vi "程序选择.vi"() -> ()   [LabVIEW 2018]
panel:
  in  "枚举":enum16{"LABVIEW仿真", "禁用FPGA输入", "使能FPGA输入"}(ring)
  in  "VISA resource name":refnum<visa-resource-name> caption="串口选择"
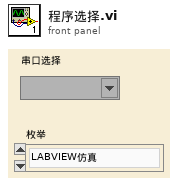
[diagram p1: front panel]
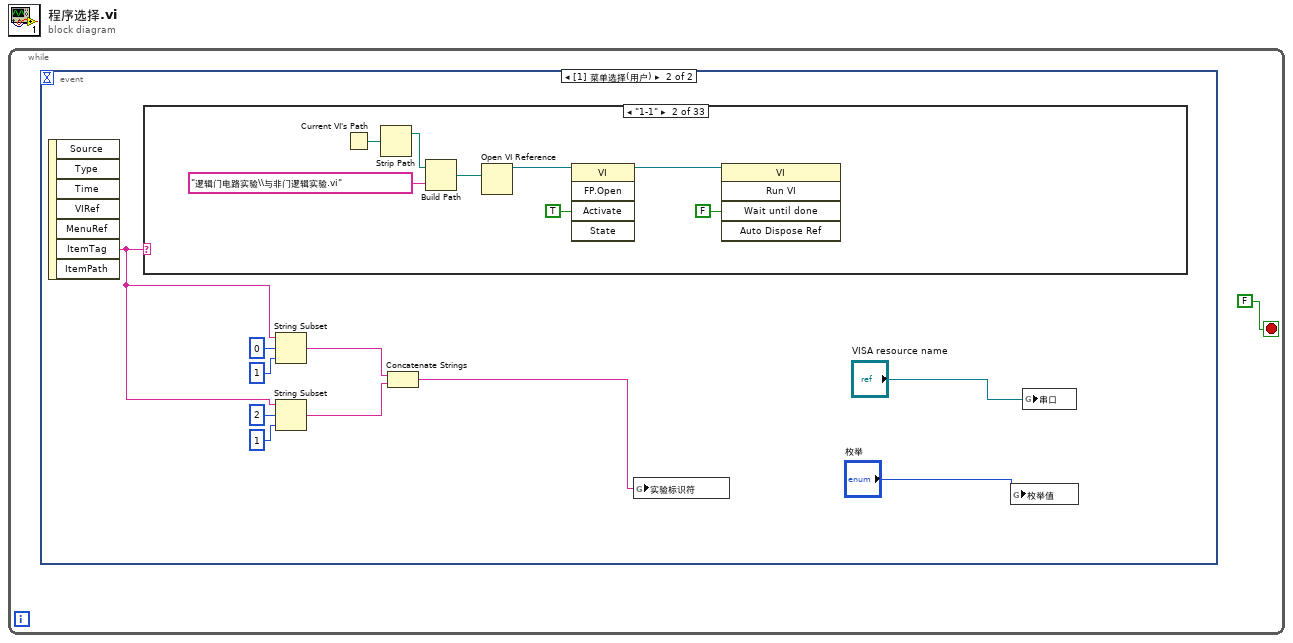
[diagram p0: block diagram]
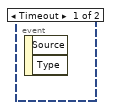
[diagram p2: hidden frame]
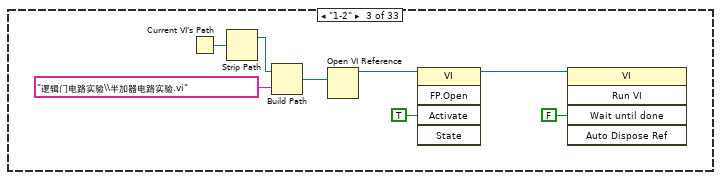
[diagram p4: hidden frame]
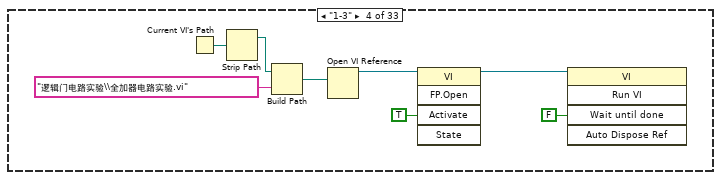
[diagram p5: hidden frame]
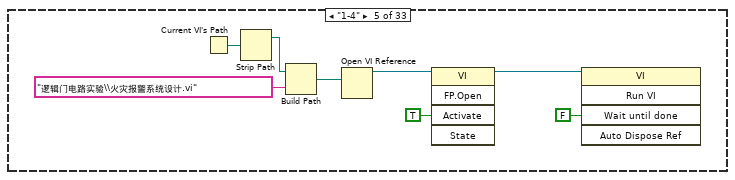
[diagram p6: hidden frame]
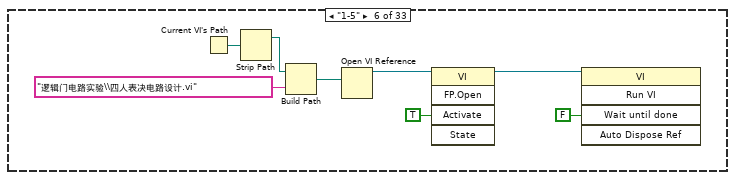
[diagram p7: hidden frame]
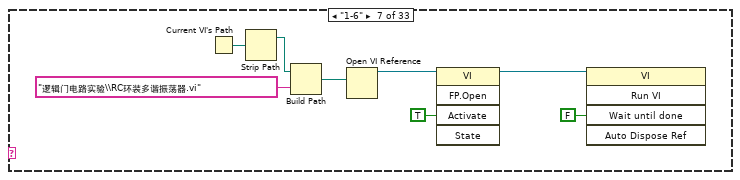
[diagram p8: hidden frame]
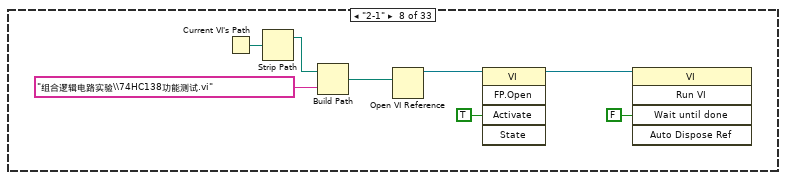
[diagram p9: hidden frame]
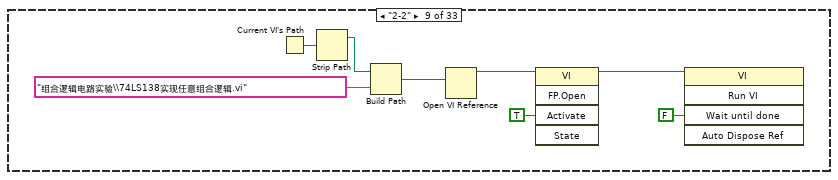
[diagram p10: hidden frame]
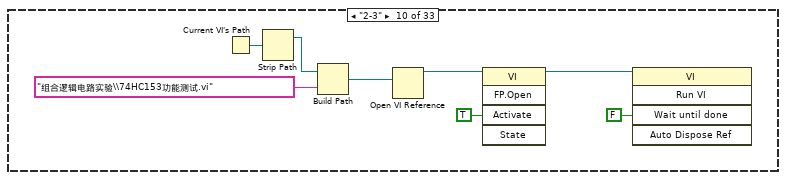
[diagram p11: hidden frame]
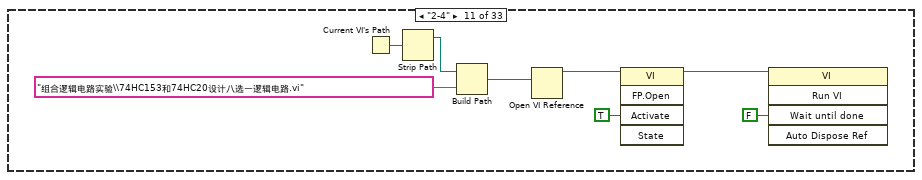
[diagram p12: hidden frame]
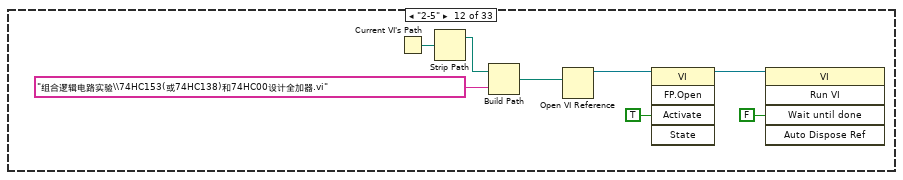
[diagram p13: hidden frame]
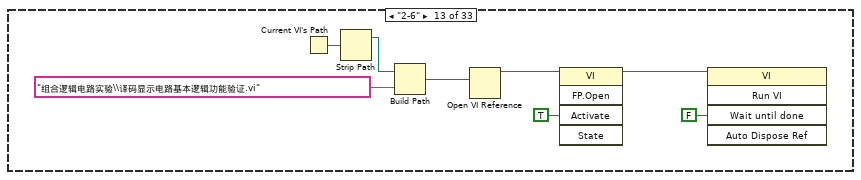
[diagram p14: hidden frame]
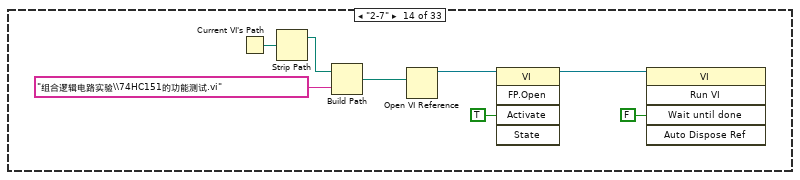
[diagram p15: hidden frame]
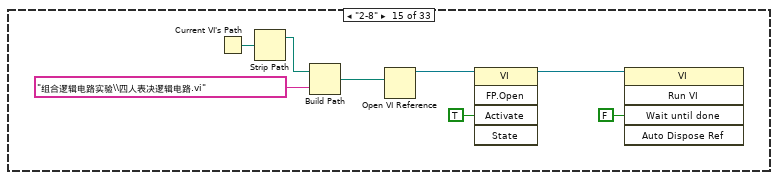
[diagram p16: hidden frame]
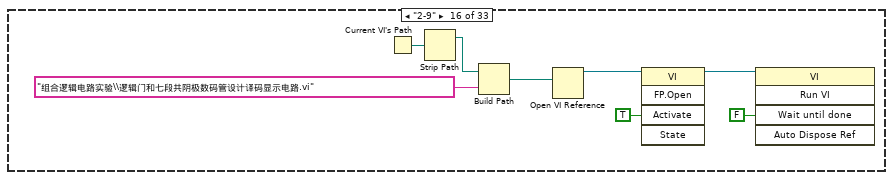
[diagram p17: hidden frame]
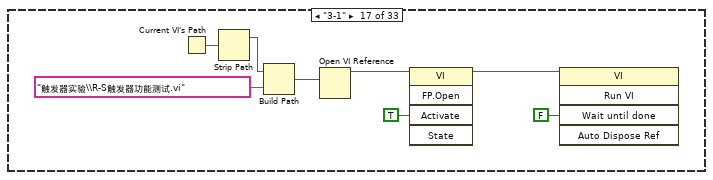
[diagram p18: hidden frame]
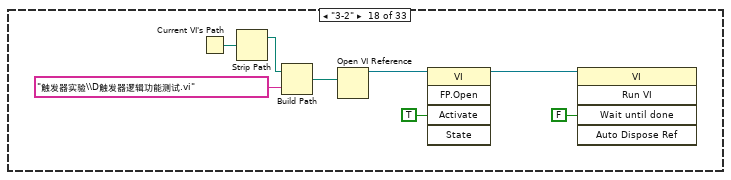
[diagram p19: hidden frame]
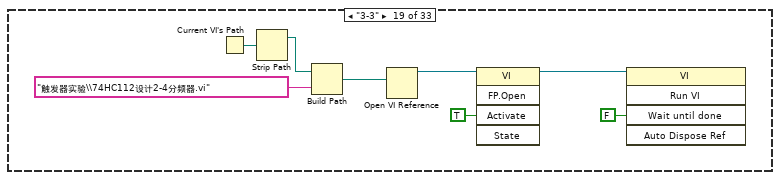
[diagram p20: hidden frame]
diagram:
  n1 = while {
    stop <- FALSE stop-if-true
    n2 = event shown="[1] 菜单选择(用户)" {
      selector: _ -> [_ _]
      dyn-events: _ -> [_ _]
      timeout: _ -> [_ _]
      event Timeout {
        n3 = event-data() -> ()  [unwired: 1 in, 2 out]
      }
      event Menu Selection (User) {
        n4 = event-data() -> ("ItemTag"=w9:string)  [unwired: 1 in, 6 out]
        n5 = case shown="\"1-1\"" w9 {
          frame "假", Default {
          }
          frame "1-1" {
            n6 = Current VI's Path() -> (path=w13:path)
            n7 = Strip Path(path=w13) -> (stripped path=w12:path)  [unwired: 1 out]
            n8 = Build Path(base path=w12, name or relative path="逻辑门电路实验\\与非门逻辑实验.vi" ("名称或相对路径")) -> (appended path=w14:path)
            n9 = Open VI Reference(vi path=w14) -> (vi reference=w19:refnum<vi>)  [unwired: 5 in, 1 out]
            n10 = invoke class="VI" method="FP.Open"(reference=w19, "Activate"=TRUE ("结束前等待")) -> (reference out=w17:refnum<vi>)  [unwired: 3 in, 4 out]
            n11 = invoke class="VI" method="Run VI"(reference=w17, "Wait until done"=FALSE ("结束前等待")) -> ()  [unwired: 3 in, 5 out]
          }
          frame "1-2" {
            n12 = Current VI's Path() -> (path=w21:path)
            n13 = Strip Path(path=w21) -> (stripped path=w20:path)  [unwired: 1 out]
            n14 = Build Path(base path=w20, name or relative path="逻辑门电路实验\\半加器电路实验.vi" ("名称或相对路径")) -> (appended path=w22:path)
            n15 = Open VI Reference(vi path=w22) -> (vi reference=w27:refnum<vi>)  [unwired: 5 in, 1 out]
            n16 = invoke class="VI" method="FP.Open"(reference=w27, "Activate"=TRUE ("结束前等待")) -> (reference out=w25:refnum<vi>)  [unwired: 3 in, 4 out]
            n17 = invoke class="VI" method="Run VI"(reference=w25, "Wait until done"=FALSE ("结束前等待")) -> ()  [unwired: 3 in, 5 out]
          }
          frame "1-3" {
            n18 = Current VI's Path() -> (path=w30:path)
            n19 = Strip Path(path=w30) -> (stripped path=w29:path)  [unwired: 1 out]
            n20 = Build Path(base path=w29, name or relative path="逻辑门电路实验\\全加器电路实验.vi" ("名称或相对路径")) -> (appended path=w28:path)
            n21 = Open VI Reference(vi path=w28) -> (vi reference=w35:refnum<vi>)  [unwired: 5 in, 1 out]
            n22 = invoke class="VI" method="FP.Open"(reference=w35, "Activate"=TRUE ("结束前等待")) -> (reference out=w33:refnum<vi>)  [unwired: 3 in, 4 out]
            n23 = invoke class="VI" method="Run VI"(reference=w33, "Wait until done"=FALSE ("结束前等待")) -> ()  [unwired: 3 in, 5 out]
          }
          frame "1-4" {
            n24 = Current VI's Path() -> (path=w38:path)
            n25 = Strip Path(path=w38) -> (stripped path=w37:path)  [unwired: 1 out]
            n26 = Build Path(base path=w37, name or relative path="逻辑门电路实验\\火灾报警系统设计.vi" ("名称或相对路径")) -> (appended path=w36:path)
            n27 = Open VI Reference(vi path=w36) -> (vi reference=w43:refnum<vi>)  [unwired: 5 in, 1 out]
            n28 = invoke class="VI" method="FP.Open"(reference=w43, "Activate"=TRUE ("结束前等待")) -> (reference out=w41:refnum<vi>)  [unwired: 3 in, 4 out]
            n29 = invoke class="VI" method="Run VI"(reference=w41, "Wait until done"=FALSE ("结束前等待")) -> ()  [unwired: 3 in, 5 out]
          }
          frame "1-5" {
            n30 = Current VI's Path() -> (path=w46:path)
            n31 = Strip Path(path=w46) -> (stripped path=w45:path)  [unwired: 1 out]
            n32 = Build Path(base path=w45, name or relative path="逻辑门电路实验\\四人表决电路设计.vi" ("名称或相对路径")) -> (appended path=w44:path)
            n33 = Open VI Reference(vi path=w44) -> (vi reference=w51:refnum<vi>)  [unwired: 5 in, 1 out]
            n34 = invoke class="VI" method="FP.Open"(reference=w51, "Activate"=TRUE ("结束前等待")) -> (reference out=w49:refnum<vi>)  [unwired: 3 in, 4 out]
            n35 = invoke class="VI" method="Run VI"(reference=w49, "Wait until done"=FALSE ("结束前等待")) -> ()  [unwired: 3 in, 5 out]
          }
          frame "1-6" {
            n36 = Current VI's Path() -> (path=w54:path)
            n37 = Strip Path(path=w54) -> (stripped path=w53:path)  [unwired: 1 out]
            n38 = Build Path(base path=w53, name or relative path="逻辑门电路实验\\RC环装多谐振荡器.vi" ("名称或相对路径")) -> (appended path=w52:path)
            n39 = Open VI Reference(vi path=w52) -> (vi reference=w59:refnum<vi>)  [unwired: 5 in, 1 out]
            n40 = invoke class="VI" method="FP.Open"(reference=w59, "Activate"=TRUE ("结束前等待")) -> (reference out=w57:refnum<vi>)  [unwired: 3 in, 4 out]
            n41 = invoke class="VI" method="Run VI"(reference=w57, "Wait until done"=FALSE ("结束前等待")) -> ()  [unwired: 3 in, 5 out]
          }
          frame "2-1" {
            n42 = Current VI's Path() -> (path=w65:path)
            n43 = Strip Path(path=w65) -> (stripped path=w66:path)  [unwired: 1 out]
            n44 = Build Path(base path=w66, name or relative path="组合逻辑电路实验\\74HC138功能测试.vi" ("名称或相对路径")) -> (appended path=w67:path)
            n45 = Open VI Reference(vi path=w67) -> (vi reference=w63:refnum<vi>)  [unwired: 5 in, 1 out]
            n46 = invoke class="VI" method="FP.Open"(reference=w63, "Activate"=TRUE ("结束前等待")) -> (reference out=w64:refnum<vi>)  [unwired: 3 in, 4 out]
            n47 = invoke class="VI" method="Run VI"(reference=w64, "Wait until done"=FALSE ("结束前等待")) -> ()  [unwired: 3 in, 5 out]
          }
          frame "2-2" {
            n48 = Current VI's Path() -> (path=w70:path)
            n49 = Strip Path(path=w70) -> (stripped path=w69:path)  [unwired: 1 out]
            n50 = Build Path(base path=w69, name or relative path="组合逻辑电路实验\\74LS138实现任意组合逻辑.vi" ("名称或相对路径")) -> (appended path=w68:path)
            n51 = Open VI Reference(vi path=w68) -> (vi reference=w75:refnum<vi>)  [unwired: 5 in, 1 out]
            n52 = invoke class="VI" method="FP.Open"(reference=w75, "Activate"=TRUE ("结束前等待")) -> (reference out=w73:refnum<vi>)  [unwired: 3 in, 4 out]
            n53 = invoke class="VI" method="Run VI"(reference=w73, "Wait until done"=FALSE ("结束前等待")) -> ()  [unwired: 3 in, 5 out]
          }
          frame "2-3" {
            n54 = Current VI's Path() -> (path=w81:path)
            n55 = Strip Path(path=w81) -> (stripped path=w82:path)  [unwired: 1 out]
            n56 = Build Path(base path=w82, name or relative path="组合逻辑电路实验\\74HC153功能测试.vi" ("名称或相对路径")) -> (appended path=w83:path)
            n57 = Open VI Reference(vi path=w83) -> (vi reference=w79:refnum<vi>)  [unwired: 5 in, 1 out]
            n58 = invoke class="VI" method="FP.Open"(reference=w79, "Activate"=TRUE ("结束前等待")) -> (reference out=w80:refnum<vi>)  [unwired: 3 in, 4 out]
            n59 = invoke class="VI" method="Run VI"(reference=w80, "Wait until done"=FALSE ("结束前等待")) -> ()  [unwired: 3 in, 5 out]
          }
          frame "2-4" {
            n60 = Current VI's Path() -> (path=w86:path)
            n61 = Strip Path(path=w86) -> (stripped path=w85:path)  [unwired: 1 out]
            n62 = Build Path(base path=w85, name or relative path="组合逻辑电路实验\\74HC153和74HC20设计八选一逻辑电路.vi" ("名称或相对路径")) -> (appended path=w84:path)
            n63 = Open VI Reference(vi path=w84) -> (vi reference=w91:refnum<vi>)  [unwired: 5 in, 1 out]
            n64 = invoke class="VI" method="FP.Open"(reference=w91, "Activate"=TRUE ("结束前等待")) -> (reference out=w89:refnum<vi>)  [unwired: 3 in, 4 out]
            n65 = invoke class="VI" method="Run VI"(reference=w89, "Wait until done"=FALSE ("结束前等待")) -> ()  [unwired: 3 in, 5 out]
          }
          frame "2-5" {
            n66 = Current VI's Path() -> (path=w94:path)
            n67 = Strip Path(path=w94) -> (stripped path=w93:path)  [unwired: 1 out]
            n68 = Build Path(base path=w93, name or relative path="组合逻辑电路实验\\74HC153(或74HC138)和74HC00设计全加器.vi" ("名称或相对路径")) -> (appended path=w92:path)
            n69 = Open VI Reference(vi path=w92) -> (vi reference=w99:refnum<vi>)  [unwired: 5 in, 1 out]
            n70 = invoke class="VI" method="FP.Open"(reference=w99, "Activate"=TRUE ("结束前等待")) -> (reference out=w97:refnum<vi>)  [unwired: 3 in, 4 out]
            n71 = invoke class="VI" method="Run VI"(reference=w97, "Wait until done"=FALSE ("结束前等待")) -> ()  [unwired: 3 in, 5 out]
          }
          frame "2-6" {
            n72 = Current VI's Path() -> (path=w102:path)
            n73 = Strip Path(path=w102) -> (stripped path=w101:path)  [unwired: 1 out]
            n74 = Build Path(base path=w101, name or relative path="组合逻辑电路实验\\译码显示电路基本逻辑功能验证.vi" ("名称或相对路径")) -> (appended path=w100:path)
            n75 = Open VI Reference(vi path=w100) -> (vi reference=w107:refnum<vi>)  [unwired: 5 in, 1 out]
            n76 = invoke class="VI" method="FP.Open"(reference=w107, "Activate"=TRUE ("结束前等待")) -> (reference out=w105:refnum<vi>)  [unwired: 3 in, 4 out]
            n77 = invoke class="VI" method="Run VI"(reference=w105, "Wait until done"=FALSE ("结束前等待")) -> ()  [unwired: 3 in, 5 out]
          }
          frame "2-7" {
            n78 = Current VI's Path() -> (path=w110:path)
            n79 = Strip Path(path=w110) -> (stripped path=w109:path)  [unwired: 1 out]
            n80 = Build Path(base path=w109, name or relative path="组合逻辑电路实验\\74HC151的功能测试.vi" ("名称或相对路径")) -> (appended path=w108:path)
            n81 = Open VI Reference(vi path=w108) -> (vi reference=w115:refnum<vi>)  [unwired: 5 in, 1 out]
            n82 = invoke class="VI" method="FP.Open"(reference=w115, "Activate"=TRUE ("结束前等待")) -> (reference out=w113:refnum<vi>)  [unwired: 3 in, 4 out]
            n83 = invoke class="VI" method="Run VI"(reference=w113, "Wait until done"=FALSE ("结束前等待")) -> ()  [unwired: 3 in, 5 out]
          }
          frame "2-8" {
            n84 = Current VI's Path() -> (path=w118:path)
            n85 = Strip Path(path=w118) -> (stripped path=w117:path)  [unwired: 1 out]
            n86 = Build Path(base path=w117, name or relative path="组合逻辑电路实验\\四人表决逻辑电路.vi" ("名称或相对路径")) -> (appended path=w116:path)
            n87 = Open VI Reference(vi path=w116) -> (vi reference=w123:refnum<vi>)  [unwired: 5 in, 1 out]
            n88 = invoke class="VI" method="FP.Open"(reference=w123, "Activate"=TRUE ("结束前等待")) -> (reference out=w121:refnum<vi>)  [unwired: 3 in, 4 out]
            n89 = invoke class="VI" method="Run VI"(reference=w121, "Wait until done"=FALSE ("结束前等待")) -> ()  [unwired: 3 in, 5 out]
          }
          frame "2-9" {
            n90 = Current VI's Path() -> (path=w126:path)
            n91 = Strip Path(path=w126) -> (stripped path=w125:path)  [unwired: 1 out]
            n92 = Build Path(base path=w125, name or relative path="组合逻辑电路实验\\逻辑门和七段共阴极数码管设计译码显示电路.vi" ("名称或相对路径")) -> (appended path=w124:path)
            n93 = Open VI Reference(vi path=w124) -> (vi reference=w131:refnum<vi>)  [unwired: 5 in, 1 out]
            n94 = invoke class="VI" method="FP.Open"(reference=w131, "Activate"=TRUE ("结束前等待")) -> (reference out=w129:refnum<vi>)  [unwired: 3 in, 4 out]
            n95 = invoke class="VI" method="Run VI"(reference=w129, "Wait until done"=FALSE ("结束前等待")) -> ()  [unwired: 3 in, 5 out]
          }
          frame "3-1" {
            n96 = Current VI's Path() -> (path=w134:path)
            n97 = Strip Path(path=w134) -> (stripped path=w133:path)  [unwired: 1 out]
            n98 = Build Path(base path=w133, name or relative path="触发器实验\\R-S触发器功能测试.vi" ("名称或相对路径")) -> (appended path=w132:path)
            n99 = Open VI Reference(vi path=w132) -> (vi reference=w139:refnum<vi>)  [unwired: 5 in, 1 out]
            n100 = invoke class="VI" method="FP.Open"(reference=w139, "Activate"=TRUE ("结束前等待")) -> (reference out=w137:refnum<vi>)  [unwired: 3 in, 4 out]
            n101 = invoke class="VI" method="Run VI"(reference=w137, "Wait until done"=FALSE ("结束前等待")) -> ()  [unwired: 3 in, 5 out]
          }
          frame "3-2" {
            n102 = Current VI's Path() -> (path=w142:path)
            n103 = Strip Path(path=w142) -> (stripped path=w141:path)  [unwired: 1 out]
            n104 = Build Path(base path=w141, name or relative path="触发器实验\\D触发器逻辑功能测试.vi" ("名称或相对路径")) -> (appended path=w140:path)
            n105 = Open VI Reference(vi path=w140) -> (vi reference=w147:refnum<vi>)  [unwired: 5 in, 1 out]
            n106 = invoke class="VI" method="FP.Open"(reference=w147, "Activate"=TRUE ("结束前等待")) -> (reference out=w145:refnum<vi>)  [unwired: 3 in, 4 out]
            n107 = invoke class="VI" method="Run VI"(reference=w145, "Wait until done"=FALSE ("结束前等待")) -> ()  [unwired: 3 in, 5 out]
          }
          frame "3-3" {
            n108 = Current VI's Path() -> (path=w150:path)
            n109 = Strip Path(path=w150) -> (stripped path=w149:path)  [unwired: 1 out]
            n110 = Build Path(base path=w149, name or relative path="触发器实验\\74HC112设计2-4分频器.vi" ("名称或相对路径")) -> (appended path=w148:path)
            n111 = Open VI Reference(vi path=w148) -> (vi reference=w155:refnum<vi>)  [unwired: 5 in, 1 out]
            n112 = invoke class="VI" method="FP.Open"(reference=w155, "Activate"=TRUE ("结束前等待")) -> (reference out=w153:refnum<vi>)  [unwired: 3 in, 4 out]
            n113 = invoke class="VI" method="Run VI"(reference=w153, "Wait until done"=FALSE ("结束前等待")) -> ()  [unwired: 3 in, 5 out]
          }
          frame "3-4" {
            n114 = Current VI's Path() -> (path=w158:path)
            n115 = Strip Path(path=w158) -> (stripped path=w157:path)  [unwired: 1 out]
            n116 = Build Path(base path=w157, name or relative path="触发器实验\\JK触发器逻辑功能的测试.vi" ("名称或相对路径")) -> (appended path=w156:path)
            n117 = Open VI Reference(vi path=w156) -> (vi reference=w163:refnum<vi>)  [unwired: 5 in, 1 out]
            n118 = invoke class="VI" method="FP.Open"(reference=w163, "Activate"=TRUE ("结束前等待")) -> (reference out=w161:refnum<vi>)  [unwired: 3 in, 4 out]
            n119 = invoke class="VI" method="Run VI"(reference=w161, "Wait until done"=FALSE ("结束前等待")) -> ()  [unwired: 3 in, 5 out]
          }
          frame "3-5" {
            n120 = Current VI's Path() -> (path=w166:path)
            n121 = Strip Path(path=w166) -> (stripped path=w165:path)  [unwired: 1 out]
            n122 = Build Path(base path=w165, name or relative path="触发器实验\\利用74HC74设计2-4分频器.vi" ("名称或相对路径")) -> (appended path=w164:path)
            n123 = Open VI Reference(vi path=w164) -> (vi reference=w171:refnum<vi>)  [unwired: 5 in, 1 out]
            n124 = invoke class="VI" method="FP.Open"(reference=w171, "Activate"=TRUE ("结束前等待")) -> (reference out=w169:refnum<vi>)  [unwired: 3 in, 4 out]
            n125 = invoke class="VI" method="Run VI"(reference=w169, "Wait until done"=FALSE ("结束前等待")) -> ()  [unwired: 3 in, 5 out]
          }
          frame "3-6" {
            n126 = Current VI's Path() -> (path=w174:path)
            n127 = Strip Path(path=w174) -> (stripped path=w173:path)  [unwired: 1 out]
            n128 = Build Path(base path=w173, name or relative path="触发器实验\\D触发器设计四人抢答电路.vi" ("名称或相对路径")) -> (appended path=w172:path)
            n129 = Open VI Reference(vi path=w172) -> (vi reference=w179:refnum<vi>)  [unwired: 5 in, 1 out]
            n130 = invoke class="VI" method="FP.Open"(reference=w179, "Activate"=TRUE ("结束前等待")) -> (reference out=w177:refnum<vi>)  [unwired: 3 in, 4 out]
            n131 = invoke class="VI" method="Run VI"(reference=w177, "Wait until done"=FALSE ("结束前等待")) -> ()  [unwired: 3 in, 5 out]
          }
          frame "4-1" {
            n132 = Current VI's Path() -> (path=w182:path)
            n133 = Strip Path(path=w182) -> (stripped path=w181:path)  [unwired: 1 out]
            n134 = Build Path(base path=w181, name or relative path="时序逻辑电路实验\\十进制同步加法计数器74HC162的功能测试.vi" ("名称或相对路径")) -> (appended path=w180:path)
            n135 = Open VI Reference(vi path=w180) -> (vi reference=w187:refnum<vi>)  [unwired: 5 in, 1 out]
            n136 = invoke class="VI" method="FP.Open"(reference=w187, "Activate"=TRUE ("结束前等待")) -> (reference out=w185:refnum<vi>)  [unwired: 3 in, 4 out]
            n137 = invoke class="VI" method="Run VI"(reference=w185, "Wait until done"=FALSE ("结束前等待")) -> ()  [unwired: 3 in, 5 out]
          }
          frame "4-2" {
            n138 = Current VI's Path() -> (path=w190:path)
            n139 = Strip Path(path=w190) -> (stripped path=w189:path)  [unwired: 1 out]
            n140 = Build Path(base path=w189, name or relative path="时序逻辑电路实验\\74HC162设计一个五进制计数器.vi" ("名称或相对路径")) -> (appended path=w188:path)
            n141 = Open VI Reference(vi path=w188) -> (vi reference=w195:refnum<vi>)  [unwired: 5 in, 1 out]
            n142 = invoke class="VI" method="FP.Open"(reference=w195, "Activate"=TRUE ("结束前等待")) -> (reference out=w193:refnum<vi>)  [unwired: 3 in, 4 out]
            n143 = invoke class="VI" method="Run VI"(reference=w193, "Wait until done"=FALSE ("结束前等待")) -> ()  [unwired: 3 in, 5 out]
          }
          frame "4-3" {
            n144 = Current VI's Path() -> (path=w198:path)
            n145 = Strip Path(path=w198) -> (stripped path=w197:path)  [unwired: 1 out]
            n146 = Build Path(base path=w197, name or relative path="时序逻辑电路实验\\两片74HC162设计一个二十四进制计数器.vi" ("名称或相对路径")) -> (appended path=w196:path)
            n147 = Open VI Reference(vi path=w196) -> (vi reference=w203:refnum<vi>)  [unwired: 5 in, 1 out]
            n148 = invoke class="VI" method="FP.Open"(reference=w203, "Activate"=TRUE ("结束前等待")) -> (reference out=w201:refnum<vi>)  [unwired: 3 in, 4 out]
            n149 = invoke class="VI" method="Run VI"(reference=w201, "Wait until done"=FALSE ("结束前等待")) -> ()  [unwired: 3 in, 5 out]
          }
          frame "4-4" {
            n150 = Current VI's Path() -> (path=w206:path)
            n151 = Strip Path(path=w206) -> (stripped path=w205:path)  [unwired: 1 out]
            n152 = Build Path(base path=w205, name or relative path="时序逻辑电路实验\\四位双向移位寄存器74HC194功能的测试.vi" ("名称或相对路径")) -> (appended path=w204:path)
            n153 = Open VI Reference(vi path=w204) -> (vi reference=w211:refnum<vi>)  [unwired: 5 in, 1 out]
            n154 = invoke class="VI" method="FP.Open"(reference=w211, "Activate"=TRUE ("结束前等待")) -> (reference out=w209:refnum<vi>)  [unwired: 3 in, 4 out]
            n155 = invoke class="VI" method="Run VI"(reference=w209, "Wait until done"=FALSE ("结束前等待")) -> ()  [unwired: 3 in, 5 out]
          }
          frame "4-5" {
            n156 = Current VI's Path() -> (path=w214:path)
            n157 = Strip Path(path=w214) -> (stripped path=w213:path)  [unwired: 1 out]
            n158 = Build Path(base path=w213, name or relative path="时序逻辑电路实验\\循环移位器.vi" ("名称或相对路径")) -> (appended path=w212:path)
            n159 = Open VI Reference(vi path=w212) -> (vi reference=w219:refnum<vi>)  [unwired: 5 in, 1 out]
            n160 = invoke class="VI" method="FP.Open"(reference=w219, "Activate"=TRUE ("结束前等待")) -> (reference out=w217:refnum<vi>)  [unwired: 3 in, 4 out]
            n161 = invoke class="VI" method="Run VI"(reference=w217, "Wait until done"=FALSE ("结束前等待")) -> ()  [unwired: 3 in, 5 out]
          }
          frame "4-6" {
            n162 = Current VI's Path() -> (path=w222:path)
            n163 = Strip Path(path=w222) -> (stripped path=w221:path)  [unwired: 1 out]
            n164 = Build Path(base path=w221, name or relative path="时序逻辑电路实验\\两片74HC194的构成八位双向移位寄存器.vi" ("名称或相对路径")) -> (appended path=w220:path)
            n165 = Open VI Reference(vi path=w220) -> (vi reference=w227:refnum<vi>)  [unwired: 5 in, 1 out]
            n166 = invoke class="VI" method="FP.Open"(reference=w227, "Activate"=TRUE ("结束前等待")) -> (reference out=w225:refnum<vi>)  [unwired: 3 in, 4 out]
            n167 = invoke class="VI" method="Run VI"(reference=w225, "Wait until done"=FALSE ("结束前等待")) -> ()  [unwired: 3 in, 5 out]
          }
          frame "5-1" {
            n168 = Current VI's Path() -> (path=w230:path)
            n169 = Strip Path(path=w230) -> (stripped path=w229:path)  [unwired: 1 out]
            n170 = Build Path(base path=w229, name or relative path="555定时器实验\\555集成定时器组成单稳态触发器.vi" ("名称或相对路径")) -> (appended path=w228:path)
            n171 = Open VI Reference(vi path=w228) -> (vi reference=w235:refnum<vi>)  [unwired: 5 in, 1 out]
            n172 = invoke class="VI" method="FP.Open"(reference=w235, "Activate"=TRUE ("结束前等待")) -> (reference out=w233:refnum<vi>)  [unwired: 3 in, 4 out]
            n173 = invoke class="VI" method="Run VI"(reference=w233, "Wait until done"=FALSE ("结束前等待")) -> ()  [unwired: 3 in, 5 out]
          }
          frame "5-2" {
            n174 = Current VI's Path() -> (path=w238:path)
            n175 = Strip Path(path=w238) -> (stripped path=w237:path)  [unwired: 1 out]
            n176 = Build Path(base path=w237, name or relative path="555定时器实验\\555集成定时器组成多谐振荡器.vi" ("名称或相对路径")) -> (appended path=w236:path)
            n177 = Open VI Reference(vi path=w236) -> (vi reference=w243:refnum<vi>)  [unwired: 5 in, 1 out]
            n178 = invoke class="VI" method="FP.Open"(reference=w243, "Activate"=TRUE ("结束前等待")) -> (reference out=w241:refnum<vi>)  [unwired: 3 in, 4 out]
            n179 = invoke class="VI" method="Run VI"(reference=w241, "Wait until done"=FALSE ("结束前等待")) -> ()  [unwired: 3 in, 5 out]
          }
          frame "5-3" {
            n180 = Current VI's Path() -> (path=w246:path)
            n181 = Strip Path(path=w246) -> (stripped path=w245:path)  [unwired: 1 out]
            n182 = Build Path(base path=w245, name or relative path="555定时器实验\\压控振荡电路.vi" ("名称或相对路径")) -> (appended path=w244:path)
            n183 = Open VI Reference(vi path=w244) -> (vi reference=w251:refnum<vi>)  [unwired: 5 in, 1 out]
            n184 = invoke class="VI" method="FP.Open"(reference=w251, "Activate"=TRUE ("结束前等待")) -> (reference out=w249:refnum<vi>)  [unwired: 3 in, 4 out]
            n185 = invoke class="VI" method="Run VI"(reference=w249, "Wait until done"=FALSE ("结束前等待")) -> ()  [unwired: 3 in, 5 out]
          }
          frame "5-4" {
            n186 = Current VI's Path() -> (path=w254:path)
            n187 = Strip Path(path=w254) -> (stripped path=w253:path)  [unwired: 1 out]
            n188 = Build Path(base path=w253, name or relative path="555定时器实验\\模拟警笛声电路.vi" ("名称或相对路径")) -> (appended path=w252:path)
            n189 = Open VI Reference(vi path=w252) -> (vi reference=w259:refnum<vi>)  [unwired: 5 in, 1 out]
            n190 = invoke class="VI" method="FP.Open"(reference=w259, "Activate"=TRUE ("结束前等待")) -> (reference out=w257:refnum<vi>)  [unwired: 3 in, 4 out]
            n191 = invoke class="VI" method="Run VI"(reference=w257, "Wait until done"=FALSE ("结束前等待")) -> ()  [unwired: 3 in, 5 out]
          }
          frame "5-5" {
            n192 = Current VI's Path() -> (path=w262:path)
            n193 = Strip Path(path=w262) -> (stripped path=w261:path)  [unwired: 1 out]
            n194 = Build Path(base path=w261, name or relative path="555定时器实验\\555组成施密特电路.vi" ("名称或相对路径")) -> (appended path=w260:path)
            n195 = Open VI Reference(vi path=w260) -> (vi reference=w267:refnum<vi>)  [unwired: 5 in, 1 out]
            n196 = invoke class="VI" method="FP.Open"(reference=w267, "Activate"=TRUE ("结束前等待")) -> (reference out=w265:refnum<vi>)  [unwired: 3 in, 4 out]
            n197 = invoke class="VI" method="Run VI"(reference=w265, "Wait until done"=FALSE ("结束前等待")) -> ()  [unwired: 3 in, 5 out]
          }
        }
        n198 = String Subset(string=w9, offset (0)=0, length (rest)=1) -> (substring=w4:string)
        n199 = String Subset(string=w9, offset (0)=2, length (rest)=1) -> (substring=w3:string)
        n200 = Concatenate Strings(w4, w3) -> (w2:string)
        n201 = global write "全局变量.vi" "实验标识符"(w2) -> ()
        n202 = global write "全局变量.vi" "枚举值"("枚举") -> ()
        n203 = global write "全局变量.vi" "串口"("VISA resource name") -> ()
      }
    }
  }
